vi "delete_selected_spots.vi"(4 "Selection/Group 3":T3[](array[typedef]), 7 "Spots 3":T1[](array[typedef]) {"Amplitude Correction" step=0.1; "Line Trapping"."Phase Gradient" step=0.05; "Line Trapping"."Vector"."x" step=1e-06 format="%#_6p"; "Line Trapping"."Vector"."y" step=1e-06 format="%#_6p"; "Line Trapping"."Vector"."z" step=1e-06 format="%#_6p"; "NA Position"."r" step=1e-06; "NA Position"."y" step=1e-06; "NA Position"."x" step=1e-06; "Position"."z" step=1e-06; "Position"."y" step=1e-06; "Position"."x" step=1e-06; "Phase" step=0.7753; "Intensity" step=0.1}) -> (0 "Selection/Group 2":T3[](array[typedef]), 3 "Spots 2":T1[](array[typedef]) {"Amplitude Correction" step=0.1; "Line Trapping"."Phase Gradient" step=0.05; "Line Trapping"."Vector"."x" step=1e-06 format="%#_6p"; "Line Trapping"."Vector"."y" step=1e-06 format="%#_6p"; "Line Trapping"."Vector"."z" step=1e-06 format="%#_6p"; "NA Position"."r" step=1e-06; "NA Position"."y" step=1e-06; "NA Position"."x" step=1e-06; "Position"."z" step=1e-06; "Position"."y" step=1e-06; "Position"."x" step=1e-06; "Phase" step=0.7753; "Intensity" step=0.1})   [LabVIEW 2015]
uses:
  selection_element.ctl
  spot.ctl
  line_trapping.ctl
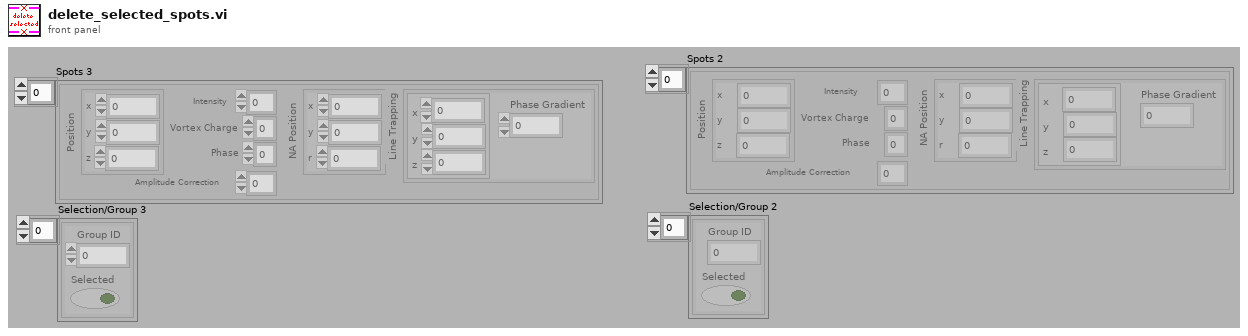
[diagram p1: front panel]
types:
  T1 = typedef "spot.ctl" = cluster{"Position":cluster{"x":dbl, "y":dbl, "z":dbl}, "Intensity":dbl, "Vortex Charge":i8, "Phase":dbl, "NA Position":cluster{"x":dbl, "y":dbl, "r":dbl}, "Line Trapping":T2, "Amplitude Correction":dbl}
  T2 = typedef "line_trapping.ctl" = cluster{"Vector":cluster{"x":dbl, "y":dbl, "z":dbl}, "Phase Gradient":dbl}
  T3 = typedef "selection_element.ctl" = cluster{"Group ID":i32, "Selected":bool}
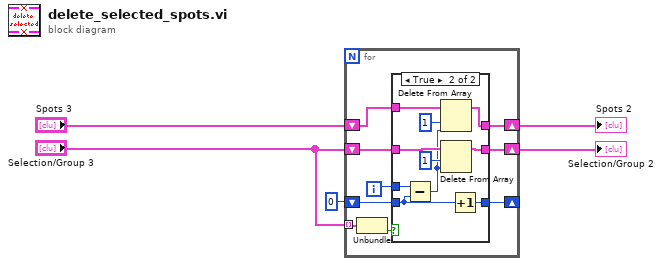
[diagram p0: block diagram]
diagram:
  n1 = for {
    tunnel: "Selection/Group 3" -> [w14] mode=indexing
    shift-right: [w12] -> w3
    shift-left: "Spots 3" -> [w13]
    shift-right: [w10] -> w4
    shift-left: "Selection/Group 3" -> [w11]
    shift-right: [w7] -> _
    shift-left: 0 ("length") -> [w8]
    i -> [w6]
    n2 = Unbundle(w14) -> ("Selected"=w9:bool)  [unwired: 1 out]
    n3 = case shown="True" w9 {
      tunnel: w13 -> [w17 w27]
      tunnel: [w17 w25] -> w12
      tunnel: w11 -> [w16 w23]
      tunnel: [w16 w22] -> w10
      tunnel: w8 -> [w15 w19]
      tunnel: [w15 w21] -> w7
      tunnel: w6 -> [_ w20]
      frame False {
      }
      frame True {
        n4 = Subtract(x=w20, y=w19) -> (x-y=w18:i32)
        n5 = Delete From Array(array=w27, length=1, index=w18) -> (array with subset deleted=w25:T1[])  [unwired: 1 out]
        n6 = Delete From Array(array=w23, length=1, index=w18) -> (array with subset deleted=w22:T3[])  [unwired: 1 out]
        n7 = Increment(x=w19) -> (x+1=w21:i32)
      }
    }
  }
  "Selection/Group 2" <- w4
  "Spots 2" <- w3
